vi "Noise-Compute Max Level (AdvFilt).vi"(0 "Noise Params":T5, 5 "Filter XCtl":T4(xcontrol), 9 "Level":T1, 11 "error in (no error)":errorcluster, 12 "Sampling Rate (Hz)":dbl, 13 "Npts":i32) -> (6 "Max Level":dbl, 10 "Level out":T1, 15 "error out":errorcluster)   [LabVIEW 2020]
uses:
  Noise Params.ctl
  Controls/Advanced Filter XCtl/Advanced Filter XCtl.xctl
  Controls/Level XCtl/Level Data.ctl
  Controls/Level XCtl/Level Units.ctl
  <vilib>/Analysis/5stat.llb/RMS (DBL).vi
  Noise-Globals.vi
  PXI DAQ VIs/DAQ Engine VIs/PXI Globals.vi
  Utility VIs/Math VIs/Linear to dB (scalar).vi
  <vilib>/Analysis/NI_AALPro.lvlib
  Controls/Level XCtl/Level XCtl.xctl
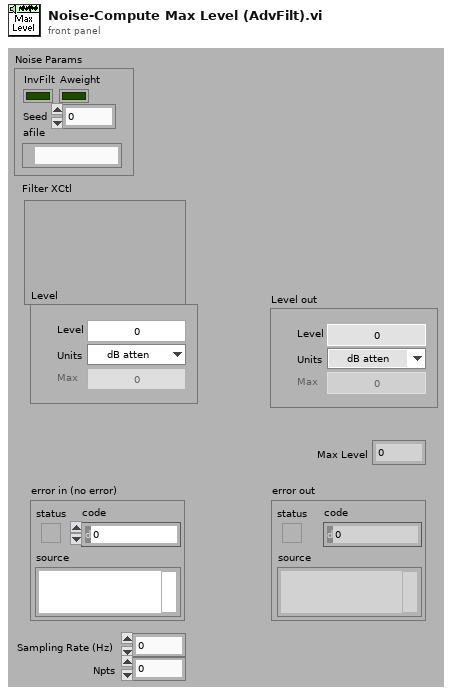
[diagram p1: front panel]
types:
  T1 = typedef "Level XCtl.xctl/Level Data.ctl" = cluster{"Level":dbl, "Units":T2, "Max":dbl, "Multiplier":dbl, "Cal File":path, "Cal":cluster{"Freq (Hz)":dbl[], "Mag (dB SPL)":dbl[], "Phase (deg)":dbl[]}}
  T2 = typedef "Level Units.ctl" = enum16{"dB atten", "dB SPL", "dB re 1 Vrms", "dB V/Hz½", "mW", "dB HL", "Volts", "dB mW"}
  T3 = typedef "Filter-Bandwidth Units.ctl" = enum16{"Linear", "Octaves", "Min-Max"}
  T4 = cluster{"Type":enum16{"Lowpass", "Highpass", "Bandpass", "Bandstop", "OFF"}, "CF (kHz)":dbl, "BW (kHz)":dbl, "Cascade":bool, "Quadrature":bool, "Scale Factor":dbl, "Stages":cluster{"IIR Filter":cluster{"filter structure":enum32{"IIR 2nd Order", "IIR 4th Order"}, "Reverse Coefficients":dbl[], "Forward Coefficients":dbl[]}, "State":dbl[]}[], "Class":enum16{"Elliptic", "Butterworth"}, "Order":i32, "BWUnits":T3}
  T5 = typedef "Noise Params.ctl" = cluster{"InvFilt":bool, "Noise":dbl[], "CurPt":i32, "Aweight":bool, "Seed":i32, "afile":path}
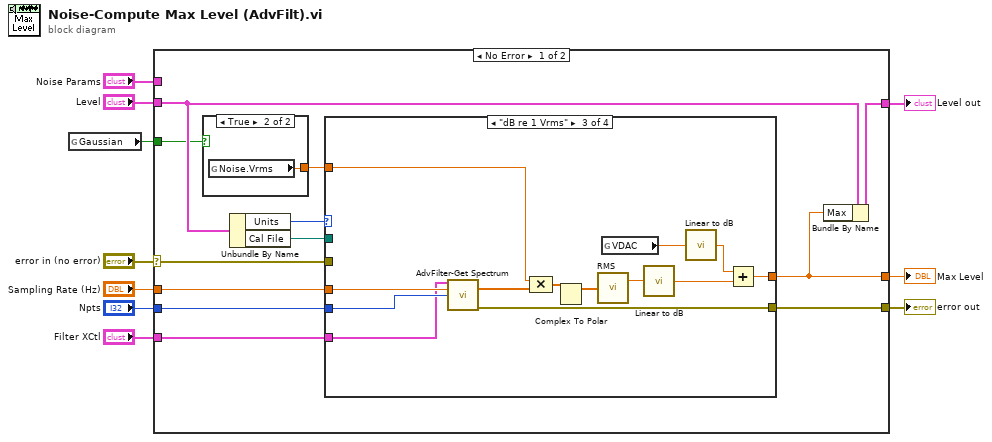
[diagram p0: block diagram]
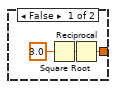
[diagram p2: hidden frame]
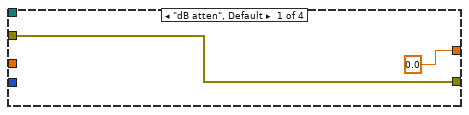
[diagram p3: hidden frame]
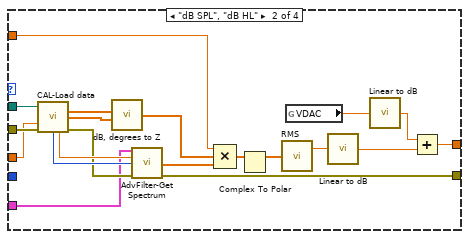
[diagram p4: hidden frame]
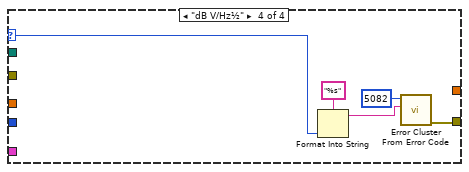
[diagram p5: hidden frame]
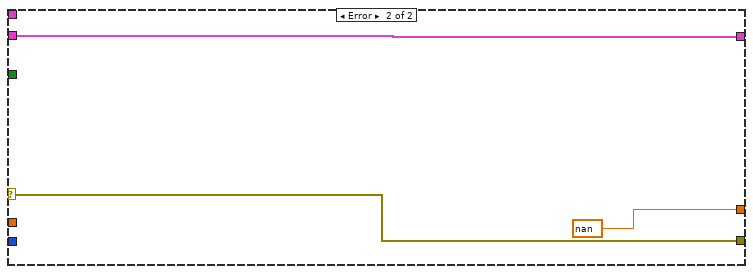
[diagram p6: hidden frame]
diagram:
  n1 = global read "Noise-Globals.vi" "Gaussian"() -> (w1:bool)
  n2 = case shown="No Error" "error in (no error)" {
    selector: "error in (no error)" -> [w22 w69]
    tunnel: "Level" -> [w17 w67]
    tunnel: "Noise Params" -> [_ _]
    tunnel: "Filter XCtl" -> [w20 _]
    tunnel: [w18 w69] -> w9
    tunnel: "Npts" -> [w21 _]
    tunnel: [w16 nan ("Reference Level")] -> w4
    tunnel: "Sampling Rate (Hz)" -> [w19 _]
    tunnel: [w15 w67] -> w2
    tunnel: w1 -> [w12 _]
    frame No Error {
      n3 = case shown="True" w12 {
        tunnel: [w25 w26] -> w13
        frame False {
          n4 = Square Root(x=3.0 ("Noise Vrms")) -> (sqrt(x)=w23:dbl)
          n5 = Reciprocal(x=w23) -> (1/x=w25:dbl)
        }
        frame True {
          n6 = global read "Noise-Globals.vi" "Noise.Vrms"() -> (w26:dbl)
        }
      }
      n7 = Unbundle By Name(w17) -> ("Units"=w14:T2, "Cal File"=w11:path)
      n8 = case shown="\"dB re 1 Vrms\"" w14 {
        selector: w14 -> [_ _ _ w62]
        tunnel: w22 -> [w27 w48 _ _]
        tunnel: w21 -> [_ _ w51 _]
        tunnel: w20 -> [_ w30 w49 _]
        tunnel: [0.0 ("Reference Level") w43 w60 _] -> w16
        tunnel: w19 -> [_ w29 w52 _]
        tunnel: [w27 w32 w53 w63] -> w18
        tunnel: w11 -> [_ w41 _ _]
        tunnel: w13 -> [_ w31 w50 _]
        frame "dB atten", Default {
        }
        frame "dB SPL", "dB HL" {
          n9 = call "CAL-Load data.vi"("user path"=w41, "Desired Fs (Hz)"=w29, "error in (no error)"=w48) -> ("Mag"=w40:dbl[], "Phase"=w39:dbl[], "npts"=w46:i32, "Fs (Hz)"=w47:dbl, "error out"=w45:errorcluster)  [unwired: 5 in, 3 out]
          n10 = call "dB, degrees to Z.vi"("Magnitude (dB)"=w40, "Phase (degrees)"=w39) -> ("Z"=w35:cdb[])  [unwired: 5 in]
          n11 = call "AdvFilter-Get Spectrum.vi"("Filter in"=w30, "Sampling Rate (Hz)"=w47, "Npts"=w46, "error in (no error)"=w45) -> ("spectrum"=w36:cdb[], "error out"=w32:errorcluster)  [unwired: 9 in, 1 out]
          n12 = Compound Arithmetic op=MULTIPLY(w31, w35, w36) -> (w37:cdb[])
          n13 = Complex To Polar(r * e^(i*theta)=w37) -> (r=w34:dbl[])  [unwired: 1 out]
          n14 = call-poly <vilib>:"RMS.vi"("X"=w34) -> ("rms value"=w38:dbl)  [unwired: 1 out]
          n15 = global read "PXI Globals.vi" "VDAC"() -> (w44:dbl)
          n16 = call-poly "Linear to dB.vi"("Linear"=w38) -> ("dB"=w33:dbl)
          n17 = call-poly "Linear to dB.vi"("Linear"=w44) -> ("dB"=w42:dbl)
          n18 = Add(x=w42, y=w33) -> (x+y=w43:dbl)
        }
        frame "dB re 1 Vrms" {
          n19 = call "AdvFilter-Get Spectrum.vi"("Filter in"=w49, "Sampling Rate (Hz)"=w52, "Npts"=w51) -> ("spectrum"=w56:cdb[], "error out"=w53:errorcluster)  [unwired: 10 in, 1 out]
          n20 = Compound Arithmetic op=MULTIPLY(w50, w56) -> (w57:cdb[])
          n21 = Complex To Polar(r * e^(i*theta)=w57) -> (r=w55:dbl[])  [unwired: 1 out]
          n22 = call-poly <vilib>:"RMS.vi"("X"=w55) -> ("rms value"=w58:dbl)  [unwired: 1 out]
          n23 = global read "PXI Globals.vi" "VDAC"() -> (w61:dbl)
          n24 = call-poly "Linear to dB.vi"("Linear"=w58) -> ("dB"=w54:dbl)
          n25 = call-poly "Linear to dB.vi"("Linear"=w61) -> ("dB"=w59:dbl)
          n26 = Add(x=w59, y=w54) -> (x+y=w60:dbl)
        }
        frame "dB V/Hz½" {
          n27 = Format Into String(format string="%s", w62) -> (resulting string=w65:string)  [unwired: 2 in, 1 out]
          n28 = call <vilib>:"Error Cluster From Error Code.vi"("error message (\"\")"=w65, "error code (0)"=5082) -> ("error out"=w63:errorcluster)  [unwired: 7 in]
        }
      }
      n29 = Bundle By Name(cluster=w17, "Max"=w16) -> (w15:T1)
    }
    frame Error {
    }
  }
  "error out" <- w9
  "Max Level" <- w4
  "Level out" <- w2
